vi "SaveSettings.vi"(11 "Settings":T1) -> ()   [LabVIEW 2020, in "DependencyChecker.lvlib"]
uses:
  <resource>/Framework/Providers/Open_GDS/DependencyViewer/DependencyChecker/DependencyChecker.lvlib
  <resource>/Framework/Providers/Open_GDS/SubVIs/GOOP_DependencySettings.ctl
  <resource>/Framework/Providers/Open_GDS/DependencyViewer/DependencyChecker/DependencyConfiguration.ctl
  <resource>/Framework/Providers/Open_GDS/DependencyViewer/DependencyChecker/FilterOptions.ctl
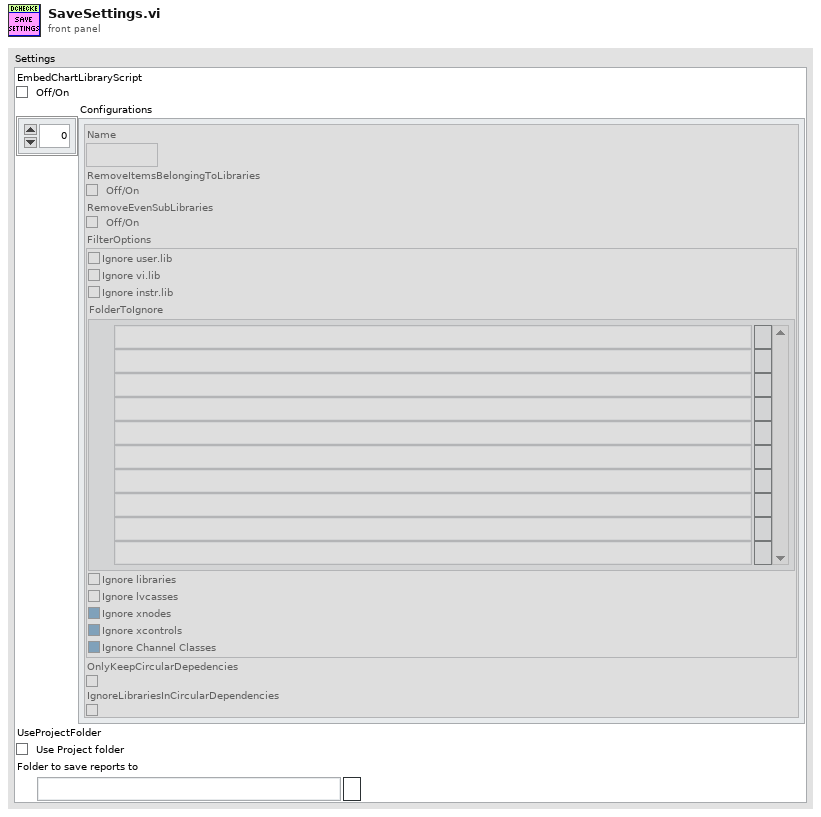
[diagram p1: front panel]
types:
  T1 = typedef "GOOP_DependencySettings.ctl" = cluster{"EmbedChartLibraryScript":bool, "Configurations":T2[], "UseProjectFolder":bool, "Folder to save reports to":path}
  T2 = typedef "DependencyChecker.lvlib/DependencyConfiguration.ctl" = cluster{"Name":string, "RemoveItemsBelongingToLibraries":bool, "RemoveEvenSubLibraries":bool, "FilterOptions":T3, "OnlyKeepCircularDepedencies":bool, "IgnoreLibrariesInCircularDependencies":bool}
  T3 = typedef "DependencyChecker.lvlib/FilterOptions.ctl" = cluster{"Ignore user.lib":bool, "Ignore vi.lib":bool, "Ignore instr.lib":bool, "FolderToIgnore":path[], "Ignore libraries":bool, "Ignore lvcasses":bool, "Ignore xnodes":bool, "Ignore xcontrols":bool, "Ignore Channel Classes":bool}
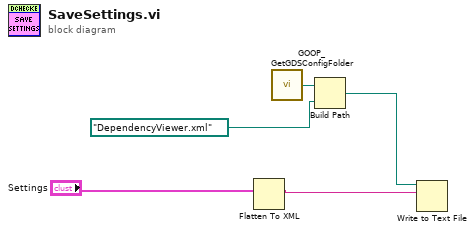
[diagram p0: block diagram]
diagram:
  n1 = Flatten To XML(6:"Settings") -> (2:w4:string)
  n2 = call <resource>:"GOOP_GetGDSConfigFolder.vi"() -> ("GDSFolderPath"=w2:path)
  n3 = Build Path(base path=w2, name or relative path=path "DependencyViewer.xml") -> (appended path=w1:path)
  n4 = Write to Text File(file (use dialog)=w1, text=w4) -> ()  [unwired: 2 in, 3 out]
